vi "Non Constant Motion 2D Motion Profile.vi"(8 "Forward?":bool, 9 "Wheel Constraints":cluster{"Vmax":dbl, "Amax":dbl}, 10 "b":dbl, 11 "Points":T2(array[cluster])) -> (0 "Total Time":dbl, 2 "Moition Profiel":T1(array[cluster]))   [LabVIEW 2016]
panel:
  in  "Vf":dbl
  in  "Vo":dbl format="%#_13g"
  out "XY Graph":cluster{dbl[], dbl[]}(graph)
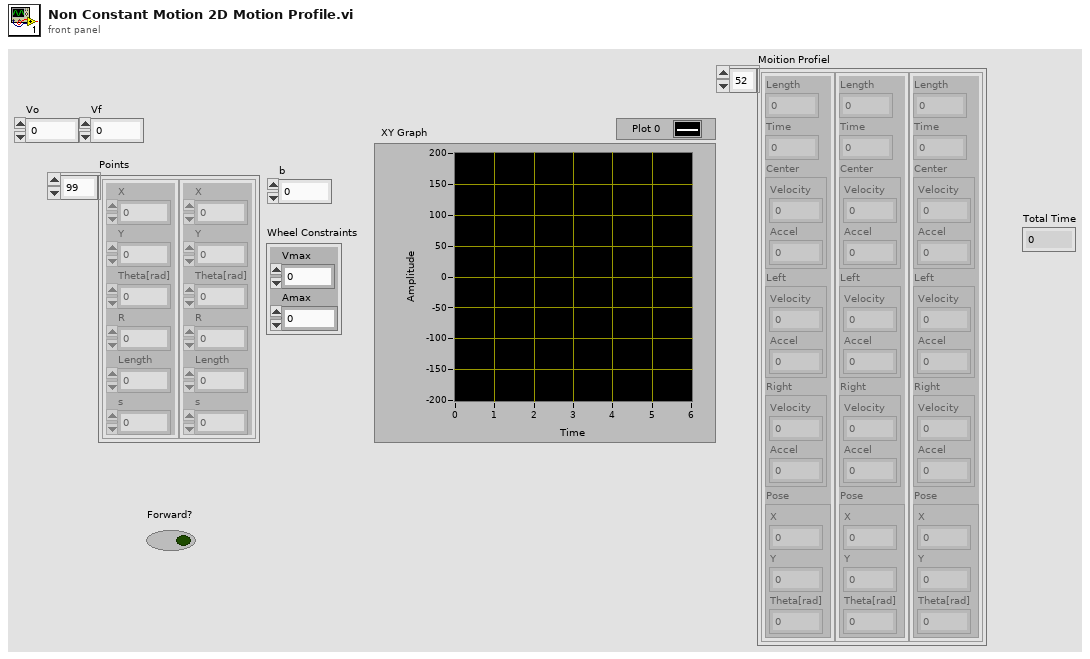
[diagram p1: front panel]
types:
  T1 = cluster{"Length":dbl, "Time":dbl, "Center":cluster{"Velocity":dbl, "Accel":dbl}, "Left":cluster{"Velocity":dbl, "Accel":dbl}, "Right":cluster{"Velocity":dbl, "Accel":dbl}, "Pose":cluster{"X":dbl, "Y":dbl, "Theta[rad]":dbl}}[]
  T2 = cluster{"X":dbl, "Y":dbl, "Theta[rad]":dbl, "R":dbl, "Length":dbl, "s":dbl}[]
  T3 = cluster{"Length":dbl, "Time":dbl, "Center":cluster{"Velocity":dbl, "Accel":dbl}, "Left":cluster{"Velocity":dbl, "Accel":dbl}, "Right":cluster{"Velocity":dbl, "Accel":dbl}, "Pose":cluster{"X":dbl, "Y":dbl, "Theta[rad]":dbl}}
  T4 = cluster{"X":dbl, "Y":dbl, "Theta[rad]":dbl, "R":dbl, "Length":dbl, "s":dbl}
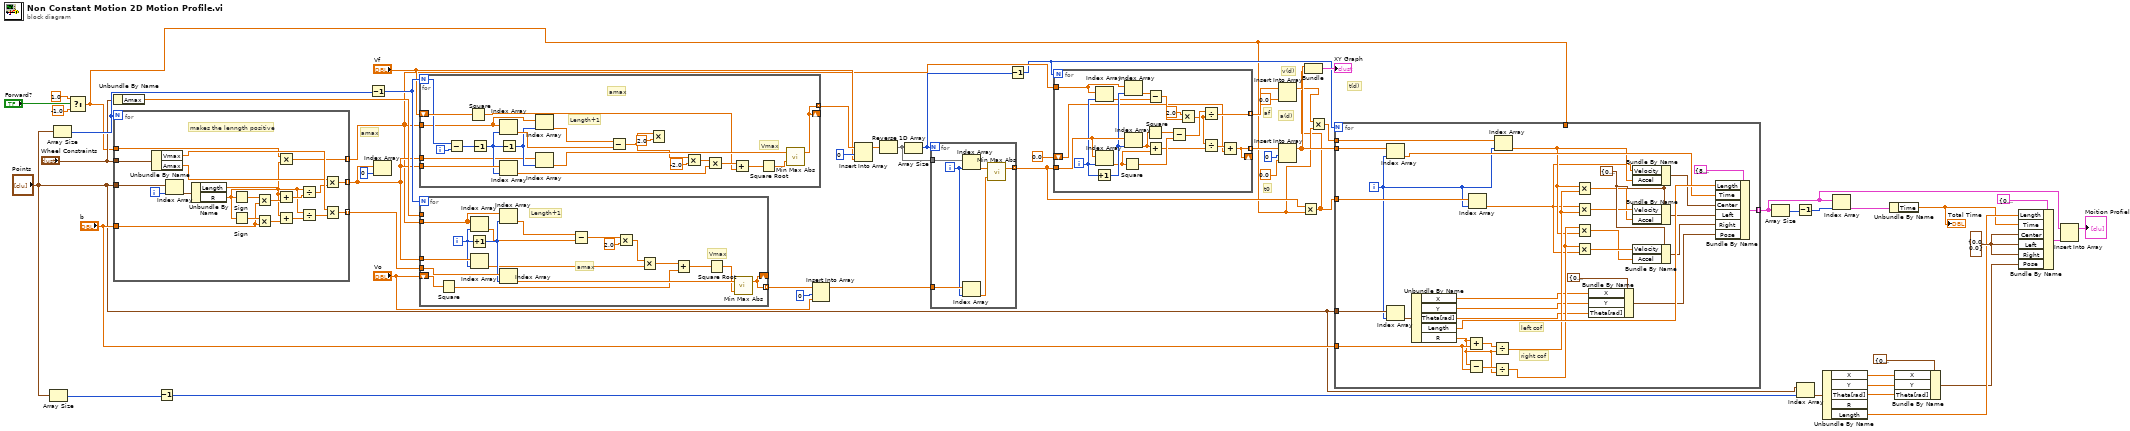
[diagram p0: block diagram]
diagram:
  w26 = cluster{"Velocity":dbl, "Accel":dbl} {"Velocity"=0.0, "Accel"=0.0} ("Center")
  # "t(d)"
  # "t0"
  # "af"
  # "a(d)"
  # "v(d)"
  # "amax"
  n1 = Array Size(array="Points") -> (size(s)=w24:i32)
  n2 = Array Size(array="Points") -> (size(s)=w55:i32)
  n3 = Select(t=1.0, s="Forward?", f=-1.0) -> (s? t:f=w3:dbl)
  n4 = Unbundle By Name("Wheel Constraints") -> ("Amax"=w42:dbl)
  n5 = for {
    N: w55 -> [_]
    tunnel: "Points" -> [w76]
    tunnel: "Wheel Constraints" -> [w72]
    tunnel: [w69] -> w54 mode=indexing
    tunnel: [w57] -> w37 mode=indexing
    tunnel: "b" -> [w62]
    tunnel: [w59] -> w40 mode=indexing
    tunnel: w3 -> [w56]
    i -> [w75]
    # "makes the lenngth positive"
    n6 = Unbundle By Name(w72) -> ("Vmax"=w70:dbl, "Amax"=w60:dbl)
    n7 = Index Array(array=w76, index=w75) -> (element=w74:T4)
    n8 = Unbundle By Name(w74) -> ("Length"=w58:dbl, "R"=w61:dbl)
    n9 = Sign(1:w61) -> (0:w65:dbl)
    n10 = Sign(1:w61) -> (0:w68:dbl)
    n11 = Multiply(x=w65, y=w62) -> (x*y=w66:dbl)
    n12 = Multiply(x=w68, y=w62) -> (x*y=w67:dbl)
    n13 = Multiply(x=w56, y=w58) -> (x*y=w57:dbl)
    n14 = Add(x=w61, y=w66) -> (x+y=w63:dbl)
    n15 = Add(x=w61, y=w67) -> (x+y=w73:dbl)
    n16 = Divide(x=w61, y=w63) -> (x/y=w64:dbl)
    n17 = Divide(x=w61, y=w73) -> (x/y=w71:dbl)
    n18 = Multiply(x=w60, y=w64) -> (x*y=w59:dbl)
    n19 = Multiply(x=w70, y=w71) -> (x*y=w69:dbl)
  }
  n20 = Decrement(x=w24) -> (x-1=w23:i32)
  n21 = Decrement(x=w55) -> (x-1=w49:i32)
  n22 = Index Array(array=w40, index=0) -> ()  [unwired: 1 out]
  n23 = for {
    N: w49 -> [w94]
    shift-right: [w83] -> _
    shift-left: "Vf" -> [w96]
    tunnel: [w83] -> w47 mode=indexing
    tunnel: w37 -> [w91]
    tunnel: w40 -> [w89]
    tunnel: w40 -> [w86]
    i -> [w93]
    # "amax"
    # "Vmax"
    # "Length+1"
    n24 = Subtract(x=w94, y=w93) -> (x-y=w92:i32)
    n25 = Square(x=w96) -> (x^2=w82:dbl)
    n26 = Decrement(x=w92) -> (x-1=w88:i32)
    n27 = Index Array(array=w91, index=w88) -> (element=w90:dbl)
    n28 = Decrement(x=w88) -> (x-1=w87:i32)
    n29 = Index Array(array=w89, index=w88) -> (element=w77:dbl)
    n30 = Index Array(array=w91, index=w87) -> (element=w78:dbl)
    n31 = Index Array(array=w86, index=w87) -> (element=w85:dbl)
    n32 = Subtract(x=w78, y=w90) -> (x-y=w79:dbl)
    n33 = Multiply(x=w79, y=2.0) -> ()  [unwired: 1 out]
    n34 = Multiply(x=w79, y=-2.0) -> (x*y=w81:dbl)
    n35 = Multiply(x=w81, y=w77) -> (x*y=w97:dbl)
    n36 = Add(x=w97, y=w82) -> (x+y=w95:dbl)
    n37 = Square Root(x=w95) -> (sqrt(x)=w84:dbl)
    n38 = call "Min Max Abs.vi"("b"=w84, "a"=w85) -> ("MinAbs(a,b)"=w83:dbl)  [unwired: 1 out]
  }
  n39 = for {
    N: w49 -> [_]
    tunnel: w37 -> [w114]
    tunnel: w54 -> [w116]
    shift-right: [w101] -> _
    shift-left: "Vo" -> [w108]
    tunnel: w42 -> [_]
    tunnel: [w101] -> w51 mode=indexing
    tunnel: w40 -> [w106]
    i -> [w105]
    # "amax"
    # "Vmax"
    # "Length+1"
    n40 = Square(x=w108) -> (x^2=w100:dbl)
    n41 = Index Array(array=w114, index=w105) -> (element=w112:dbl)
    n42 = Increment(x=w105) -> (x+1=w115:i32)
    n43 = Index Array(array=w106, index=w105) -> (element=w102:dbl)
    n44 = Index Array(array=w114, index=w115) -> (element=w113:dbl)
    n45 = Index Array(array=w116, index=w115) -> (element=w104:dbl)
    n46 = Subtract(x=w113, y=w112) -> (x-y=w111:dbl)
    n47 = Multiply(x=w111, y=2.0) -> (x*y=w99:dbl)
    n48 = Multiply(x=w99, y=w102) -> (x*y=w109:dbl)
    n49 = Add(x=w109, y=w100) -> (x+y=w107:dbl)
    n50 = Square Root(x=w107) -> (sqrt(x)=w103:dbl)
    n51 = call "Min Max Abs.vi"("b"=w103, "a"=w104) -> ("MinAbs(a,b)"=w101:dbl)  [unwired: 1 out]
  }
  n52 = Insert Into Array(array=w51, index=0, new element="Vo") -> (w43:dbl[])
  n53 = Insert Into Array(array=w47, index=0, new element="Vf") -> (w45:dbl[])
  n54 = Reverse 1D Array(array=w45) -> (reversed array=w44:dbl[])
  n55 = Array Size(array=w44) -> (size(s)=w38:i32)
  n56 = for {
    N: w38 -> [_]
    tunnel: w44 -> [w122]
    tunnel: w43 -> [w121]
    tunnel: [w118] -> w5 mode=indexing
    i -> [w117]
    n57 = Index Array(array=w122, index=w117) -> (element=w120:dbl)
    n58 = Index Array(array=w121, index=w117) -> (element=w119:dbl)
    n59 = call "Min Max Abs.vi"("b"=w119, "a"=w120) -> ("MinAbs(a,b)"=w118:dbl)  [unwired: 1 out]
  }
  n60 = Decrement(x=w38) -> (x-1=w30:i32)
  n61 = for {
    N: w30 -> [_]
    tunnel: w5 -> [w141]
    tunnel: w37 -> [w135]
    tunnel: [w131] -> w36 mode=indexing
    shift-right: [w123] -> _
    shift-left: 0.0 -> [w124]
    tunnel: [w123] -> w33 mode=indexing
    i -> [w136]
    n62 = Index Array(array=w135, index=w136) -> (element=w133:dbl)
    n63 = Index Array(array=w141, index=w136) -> (element=w130:dbl)
    n64 = Increment(x=w136) -> (x+1=w134:i32)
    n65 = Square(x=w130) -> (x^2=w138:dbl)
    n66 = Index Array(array=w135, index=w134) -> (element=w129:dbl)
    n67 = Index Array(array=w141, index=w134) -> (element=w128:dbl)
    n68 = Square(x=w128) -> (x^2=w140:dbl)
    n69 = Subtract(x=w129, y=w133) -> (x-y=w132:dbl)
    n70 = Add(x=w128, y=w130) -> (x+y=w126:dbl)
    n71 = Subtract(x=w140, y=w138) -> (x-y=w139:dbl)
    n72 = Multiply(x=2.0, y=w132) -> (x*y=w127:dbl)
    n73 = Divide(x=w139, y=w127) -> (x/y=w131:dbl)
    n74 = Divide(x=w127, y=w126) -> (x/y=w125:dbl)
    n75 = Add(x=w125, y=w124) -> (x+y=w123:dbl)
  }
  n76 = Insert Into Array(array=w36, new element=0.0 ("new element/subarray")) -> (w4:dbl[])  [unwired: 1 in]
  n77 = Insert Into Array(array=w33, index=0, new element=0.0 ("new element/subarray")) -> (w29:dbl[])
  n78 = Multiply(x=w5, y=w3) -> (x*y=w1:dbl[])
  n79 = Bundle(w29, w1) -> (→"XY Graph":cluster{dbl[], dbl[]})  [unwired: 1 in]
  n80 = Multiply(x=w4, y=w3) -> (x*y=w2:dbl[])
  n81 = for {
    N: w30 -> [_]
    tunnel: "Points" -> [w172]
    tunnel: w29 -> [w168]
    tunnel: w1 -> [w165]
    tunnel: w2 -> [w163]
    tunnel: "b" -> [w161]
    tunnel: [w143] -> w16 mode=indexing
    tunnel: w3 -> [_]
    i -> [w164]
    w158 = cluster{"Velocity":dbl, "Accel":dbl} {"Velocity"=0.0, "Accel"=0.0} ("Center")
    # "right cof"
    # "left cof"
    n82 = Index Array(array=w168, index=w164) -> (element=w167:dbl)
    n83 = Index Array(array=w172, index=w164) -> (element=w171:T4)
    n84 = Unbundle By Name(w171) -> ("X"=w147:dbl, "Y"=w146:dbl, "Theta[rad]"=w145:dbl, "Length"=w169:dbl, "R"=w159:dbl)
    n85 = Add(x=w159, y=w161) -> (x+y=w162:dbl)
    n86 = Subtract(x=w159, y=w161) -> (x-y=w160:dbl)
    n87 = Index Array(array=w165, index=w164) -> (element=w142:dbl)
    n88 = Divide(x=w162, y=w159) -> (x/y=w156:dbl)
    n89 = Divide(x=w160, y=w159) -> (x/y=w153:dbl)
    n90 = Index Array(array=w163, index=w164) -> (element=w152:dbl)
    n91 = Multiply(x=w152, y=w156) -> (x*y=w155:dbl)
    n92 = Multiply(x=w142, y=w156) -> (x*y=w157:dbl)
    n93 = Multiply(x=w153, y=w152) -> (x*y=w150:dbl)
    n94 = Multiply(x=w153, y=w142) -> (x*y=w151:dbl)
    n95 = Bundle By Name(cluster=cluster{"X":dbl, "Y":dbl, "Theta[rad]":dbl} {"X"=0.0, "Y"=0.0, "Theta[rad]"=0.0} ("Pose"), "X"=w147, "Y"=w146, "Theta[rad]"=w145) -> (w144:cluster{"X":dbl, "Y":dbl, "Theta[rad]":dbl})
    n96 = Bundle By Name(cluster=w158, "Velocity"=w142, "Accel"=w152) -> (w166:cluster{"Velocity":dbl, "Accel":dbl})
    n97 = Bundle By Name(cluster=w158, "Velocity"=w157, "Accel"=w155) -> (w154:cluster{"Velocity":dbl, "Accel":dbl})
    n98 = Bundle By Name(cluster=w158, "Velocity"=w151, "Accel"=w150) -> (w149:cluster{"Velocity":dbl, "Accel":dbl})
    n99 = Bundle By Name(cluster=T3 {"Length"=86.23328135958147, "Time"=0.5454545454545454, "Center"={"Velocity"=0.0, "Accel"=0.0}, "Left"={"Velocity"=0.0, "Accel"=0.0}, "Right"={"Velocity"=0.0, "Accel"=0.0}, "Pose"={"X"=73.70398196844478, "Y"=36.51389932381669, "Theta[rad]"=0.8460969888494012}} ("Point"), "Length"=w169, "Time"=w167, "Center"=w166, "Left"=w154, "Right"=w149, "Pose"=w144) -> (w143:T3)
  }
  n100 = Array Size(array=w16) -> (size(s)=w18:i32)
  n101 = Decrement(x=w18) -> (x-1=w17:i32)
  n102 = Index Array(array="Points", index=w23) -> (element=w22:T4)
  n103 = Unbundle By Name(w22) -> ("X"=w12:dbl, "Y"=w11:dbl, "Theta[rad]"=w10:dbl, "Length"=w21:dbl)  [unwired: 1 out]
  n104 = Index Array(array=w16, index=w17) -> (element=w15:T3)
  n105 = Unbundle By Name(w15) -> ("Time"=w14:dbl)
  "Total Time" <- w14
  n106 = Bundle By Name(cluster=cluster{"X":dbl, "Y":dbl, "Theta[rad]":dbl} {"X"=0.0, "Y"=0.0, "Theta[rad]"=0.0} ("Pose"), "X"=w12, "Y"=w11, "Theta[rad]"=w10) -> (w9:cluster{"X":dbl, "Y":dbl, "Theta[rad]":dbl})
  n107 = Bundle By Name(cluster=T3 {"Length"=0.0, "Time"=0.0, "Center"={"Velocity"=0.0, "Accel"=0.0}, "Left"={"Velocity"=0.0, "Accel"=0.0}, "Right"={"Velocity"=0.0, "Accel"=0.0}, "Pose"={"X"=0.0, "Y"=0.0, "Theta[rad]"=0.0}} ("new element/subarray"), "Length"=w21, "Time"=w14, "Center"=w26, "Left"=w26, "Right"=w26, "Pose"=w9) -> (w20:T3)
  n108 = Insert Into Array(array=w16, new element=w20) -> (→"Moition Profiel":T1)  [unwired: 1 in]
